vi "calc_focus_test.vi"() -> ()   [LabVIEW 2017]
uses:
  Vision.lvlib
panel:
  in  "File Path":path=path "C:/Users/Caleb/Desktop/obama.jpg"
  out "focus":sgl
  out "error out":errorcluster
  out "Image":T1(plugin-control)
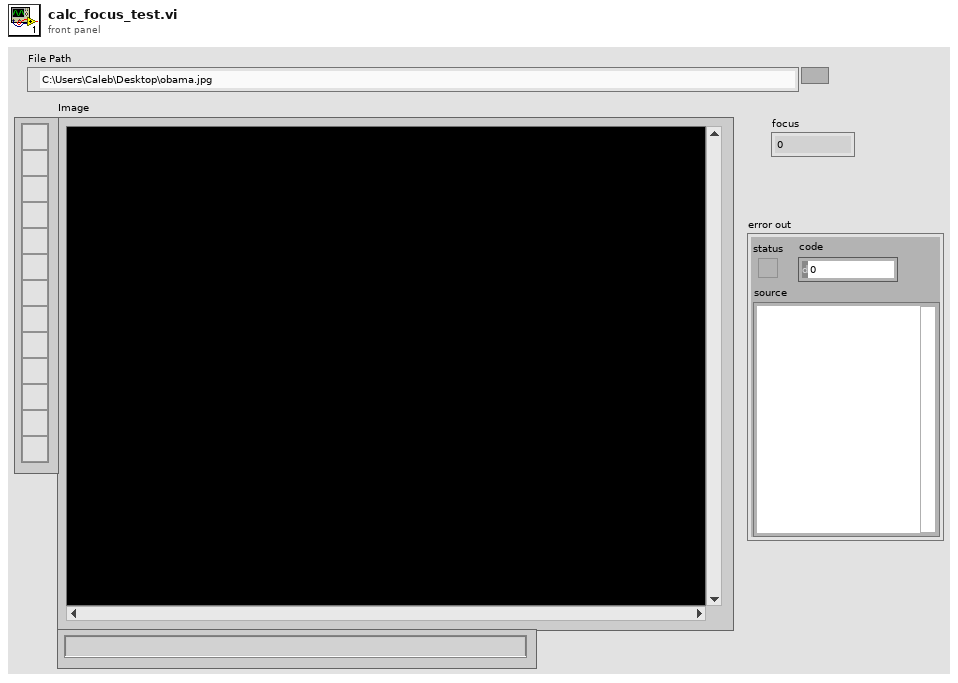
[diagram p1: front panel]
types:
  T1 = typedef "IMAQ Image.ctl" = refnum<image>
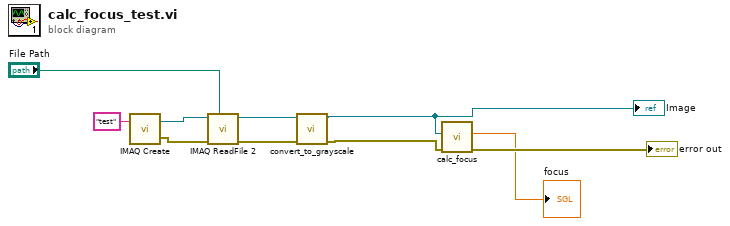
[diagram p0: block diagram]
diagram:
  n1 = call "IMAQ Create"("Image Name"="test") -> ("New Image"=w10:T1, "error out"=w8:errorcluster)  [unwired: 4 in]
  n2 = call "IMAQ ReadFile 2"("File Path"="File Path", "error in (no error)"=w8, "Image"=w10) -> ("error out"=w3:errorcluster, "Image Out"=w4:T1)  [unwired: 4 in, 3 out]
  n3 = call "convert_to_grayscale.vi"("error in (no error)"=w3, "Image in"=w4) -> ("error out"=w2:errorcluster, "Image out"=w1:T1)  [unwired: 8 in]
  "Image" <- w1
  n4 = call "calc_focus.vi"("error in"=w2, "Image"=w1) -> ("error out"=→"error out":errorcluster, "focus"=→"focus":sgl)  [unwired: 7 in, 1 out]
